vi "Port Under Mouse.vi"(8 "error in (no error)":errorcluster, 10 "point":cluster{"x":i16, "y":i16}, 11 "FSM in":refnum<class "FSM.Node.lvclass">) -> (0 "error out":errorcluster, 1 "found?":bool, 2 "Port":refnum<class "FSM.Port.lvclass">, 3 "FSM out":refnum<class "FSM.Node.lvclass">)   [LabVIEW 2015, in "FSM.Node.lvclass"]
uses:
  FSM.Node.lvclass
  FSM.Port/FSM.Port.lvclass
  FSM.Node.lvclass/FSM.Node.ctl
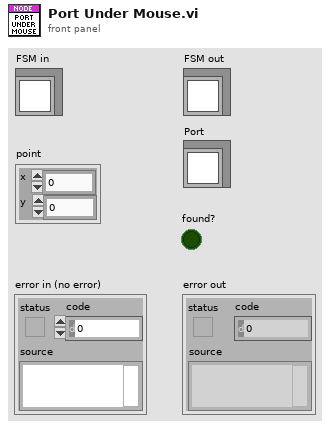
[diagram p1: front panel]
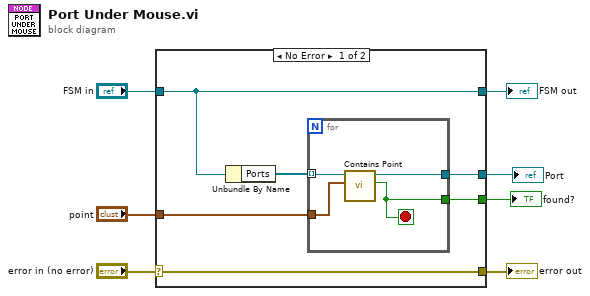
[diagram p0: block diagram]
diagram:
  n1 = case shown="No Error" "error in (no error)" {
    selector: "error in (no error)" -> [w13 w19]
    tunnel: [w13 w19] -> w6
    tunnel: [w12 w18] -> w4
    tunnel: "FSM in" -> [w12 w18]
    tunnel: "point" -> [w10 _]
    tunnel: [w9 _] -> w2
    tunnel: [w8 _] -> w1
    frame No Error {
      n2 = Unbundle By Name(w12) -> ("Ports"=w11:refnum<class "FSM.Port.lvclass">[])
      n3 = for {
        tunnel: w11 -> [w17] mode=indexing
        tunnel: w10 -> [w16]
        tunnel: [w15] -> w8
        tunnel: [w14] -> w9
        stop <- w14 stop-if-true
        n4 = call "Contains Point.vi"("point"=w16, "Port in"=w17) -> ("contains point"=w14:bool, "Port out"=w15:refnum<class "FSM.Port.lvclass">)  [unwired: 7 in, 1 out]
      }
    }
    frame Error {
    }
  }
  "error out" <- w6
  "FSM out" <- w4
  "Port" <- w1
  "found?" <- w2
